vi "Handle Received Heartbeat Message.vi"(8 "error in":errorcluster, 10 "CANopen Message":refnum<class "CANopen Response Message.lvclass">, 11 "CANopen Master in":refnum<class "CANopen Master.lvclass">) -> (0 "error out":errorcluster, 3 "CANopen Master out":refnum<class "CANopen Master.lvclass">)   [LabVIEW 2024, in "CANopen Master.lvlib" / "CANopen Master.lvclass"]
doc: "Handles a received NMT Message. Resets an awaited heartbeat. Extracts Sender's state and fires a Node Discovered event in case a new node is on the bus."
uses:
  CANopen Master.lvclass
  CANopen Master.lvclass/CANopen Master.ctl
  Network Management/Network Mangement.lvclass
  CANopen Response/CANopen Response Message.lvclass
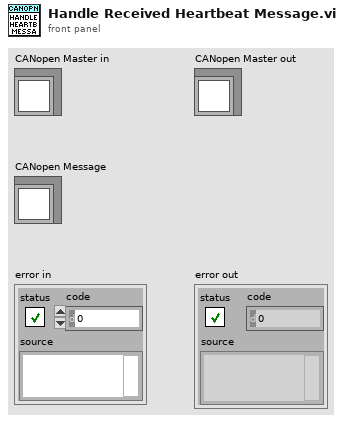
[diagram p1: front panel]
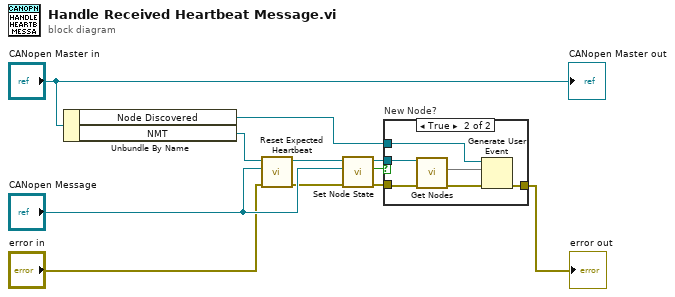
[diagram p0: block diagram]
diagram:
  n1 = Unbundle By Name("CANopen Master in") -> ("Node Discovered"=w7:refnum<user-event>, "NMT"=w5:refnum<class "Network Mangement.lvclass">)
  n2 = call "Reset Expected Heartbeat.vi"("Error In"="error in", "CANopen Message"="CANopen Message", "reference in"=w5) -> ("Error Out"=w1:errorcluster, "reference out"=w4:refnum<class "Network Mangement.lvclass">)  [unwired: 7 in]
  n3 = call "Set Node State.vi"("Error In"=w1, "CANopen Message"="CANopen Message", "reference in"=w4) -> ("Error Out"=w9:errorcluster, "New Node/State?"=w10:bool, "reference out"=w8:refnum<class "Network Mangement.lvclass">)  [unwired: 6 in]
  n4 = case "New Node?" shown="True" w10 {
    tunnel: w9 -> [w12 w17]
    tunnel: w8 -> [_ w18]
    tunnel: w7 -> [_ w15]
    tunnel: [w12 w13] -> w6
    frame False {
    }
    frame True {
      n5 = call "Get Nodes.vi"("Error In"=w17, "reference in"=w18) -> ("Error Out"=w14:errorcluster, "Nodes"=w16:map{u8, u8})  [unwired: 7 in, 1 out]
      n6 = Generate User Event(user event=w15, event data cluster=w16, error in=w14) -> (error out=w13:errorcluster)  [unwired: 1 in, 1 out]
    }
  }
  "error out" <- w6
  "CANopen Master out" <- "CANopen Master in"
